vi "Close.vi"(8 "error in":errorcluster, 11 "Current Nominal Value in":refnum<class "Current Nominal Value.lvclass">) -> (0 "error out":errorcluster, 3 "Current Nominal Value out":refnum<class "Current Nominal Value.lvclass">)   [LabVIEW 2023, in "Current Nominal Value.lvclass"]
uses:
  Current Nominal Value.lvclass
  Parents/Nominal Value/Nominal Value.lvclass
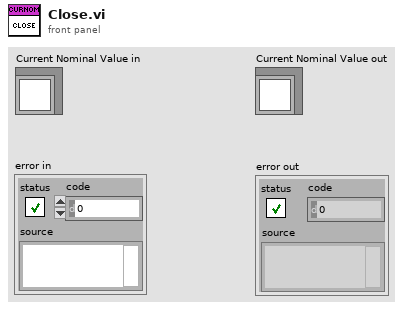
[diagram p1: front panel]
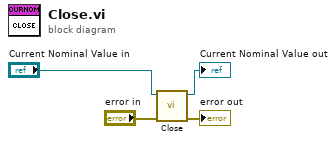
[diagram p0: block diagram]
diagram:
  n1 = call-parent "Close.vi"("error in"="error in", "Nominal Value in"="Current Nominal Value in") -> ("error out"=→"error out":errorcluster, "Nominal Value out"=→"Current Nominal Value out":refnum<class "Current Nominal Value.lvclass">)  [unwired: 8 in]
